vi "5 Table using FOR Loop.vi"() -> ()   [LabVIEW 2016]
panel:
  out "5 Table":i32[](array[numeric])
  in  "No. of Iterations":i32
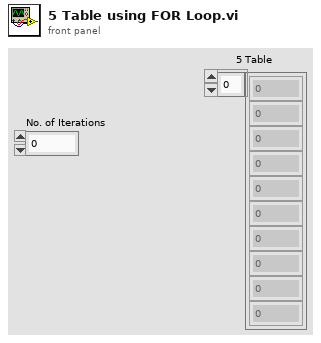
[diagram p1: front panel]
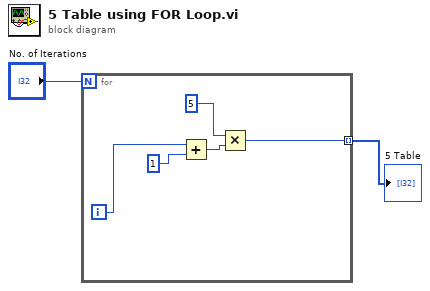
[diagram p0: block diagram]
diagram:
  n1 = for {
    N: "No. of Iterations" -> [_]
    tunnel: [w3] -> w1 mode=indexing
    i -> [w4]
    n2 = Add(x=w4, y=1) -> (x+y=w6:i32)
    n3 = Multiply(x=5, y=w6) -> (x*y=w3:i32)
  }
  "5 Table" <- w1
